vi "Logger-Purge Old Logs.vi"(0 "Folder":path, 5 "Name":string, 9 "Retain (days)":i32, 11 "error in (no error)":errorcluster) -> (15 "error out":errorcluster)   [LabVIEW 2020]
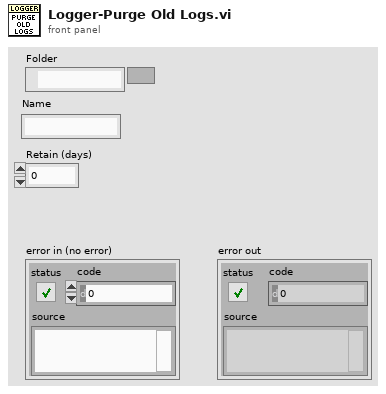
[diagram p1: front panel]
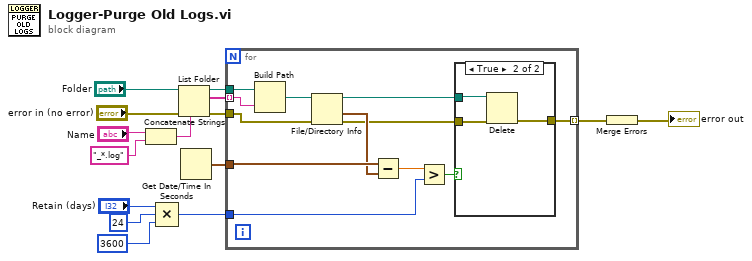
[diagram p0: block diagram]
diagram:
  n1 = Concatenate Strings("Name", "_*.log" ("string")) -> (w12:string)
  n2 = Compound Arithmetic op=MULTIPLY("Retain (days)", 24 ("value"), 3600 ("value")) -> (w1:i32)
  n3 = List Folder(path="Folder", pattern=w12, error in="error in (no error)") -> (path out=w10:path, filenames=w9:string[], error out=w7:errorcluster)  [unwired: 1 in, 1 out]
  n4 = Get Date/Time In Seconds() -> (seconds since 1Jan1904=w8:timestamp)
  n5 = for {
    tunnel: w10 -> [w27]
    tunnel: w9 -> [w26] mode=indexing
    tunnel: w8 -> [w24]
    tunnel: w7 -> [w22]
    tunnel: w1 -> [w20]
    tunnel: [w16] -> w3 mode=indexing
    n6 = Build Path(base path=w27, name or relative path=w26) -> (appended path=w25:path)
    n7 = File/Directory Info(path=w25, error in=w22) -> (path out=w18:path, last mod=w23:timestamp, error out=w17:errorcluster)  [unwired: 4 out]
    n8 = Subtract(x=w24, y=w23) -> (x-y=w21:dbl)
    n9 = Greater?(x=w21, y=w20) -> (0:w19:bool)
    n10 = case shown="True" w19 {
      tunnel: w18 -> [_ w30]
      tunnel: w17 -> [w28 w31]
      tunnel: [w28 w29] -> w16
      frame False {
      }
      frame True {
        n11 = Delete(path (use dialog)=w30, error in=w31) -> (error out=w29:errorcluster)  [unwired: 3 in, 2 out]
      }
    }
  }
  n12 = Merge Errors(w3) -> (→"error out":errorcluster)
